vi "uServices Status Check.vi"(8 "error in (no error)":errorcluster, 11 "Guardian in":refnum<class "Guardian.lvclass">) -> (0 "error out":errorcluster, 3 "Guardian out":refnum<class "Guardian.lvclass">)   [LabVIEW 2026, in "TALOS.lvlib" / "Guardian.lvlib" / "Guardian.lvclass"]
uses:
  Guardian.lvclass
  C:/LabVIEW Code/TALOS/builds/Actor Framework PPL/Actor Framework.lvlibp/1abvi3w/vi.lib/ActorFramework/Actor/Actor.lvclass
  Ancestor/Ancestor/Ancestor.lvclass/Ancestor.ctl
  Classes/Speedometer/Speedometer.lvclass/Speedometer.ctl
  Classes/uService List/uService List.lvclass/uService List.ctl
  Guardian Messages/uService not responding Msg/uService not responding Msg.lvclass/uService not responding Msg.ctl
  Classes/uService List/Get all IDs.vi
  Classes/uService List/Get Last Pat.vi
  Support VIs/Generate Error.vi
  <vilib>/Utility/High Resolution Relative Seconds.vi
  FGV/Error Memory/Get Error Description.vi
  Support VIs/Get PC name.vi
  Ancestor/Ancestor/Read ID.vi
  Support VIs/Get Class Name.vi
  FGV/Error Memory/Error Memory Core.vi
  <vilib>/AdvancedString/Delimited String to 1D String Array.vi
  <vilib>/AdvancedString/Delimited String to 1D String Array (string).vi
  Support VIs/Circus Root Path.vi
  FGV/Error Memory/Error Crt Lvl checker.vi
  FGV/Error Memory/Error Memory Core.vi/40c8088d-b597-4017-91af-faa98e00292e.vi
  FGV/Error Memory/Error Memory Core.vi/d4a3ab98-063c-4e44-b43d-fbdcfe6c2be2.vi
  Support VIs/Global Memory.vi
  <vilib>/Utility/LVClass/Get LV Class Name.vi
  Support VIs/Is in Packed Library.vi
  Support VIs/TALOS Root path.vi
  Support VIs/Read CSV worksheet.vi
  Support VIs/Global Constants.vi
  <vilib>/Utility/error.llb/General Error Handler.vi
  <vilib>/Utility/config.llb/Open Config Data.vi
  <vilib>/Utility/config.llb/Get Section Names.vi
  <vilib>/Utility/config.llb/Get Key Names.vi
  <vilib>/Utility/config.llb/Read Key.vi
  <vilib>/Utility/config.llb/Read Key (String).vi
  <vilib>/Utility/config.llb/Close Config Data.vi
  builds/Actor Framework PPL/Actor Framework.lvlibp/1abvi3w/vi.lib/ActorFramework/Message Enqueuer/Enqueue.vi
  Support VIs/Error Log.vi
  Support VIs/System Log.vi
  Ancestor/Ancestor/Ancestor.lvclass
  <vilib>/Comparison/Equal/Equal Functor/Equal Functor.lvclass
  Classes/Speedometer/Speedometer.lvclass
  Guardian Messages/uService not responding Msg/uService not responding Msg.lvclass
  TALOS.lvlib
  Classes/uService List/uService List.lvclass
  builds/Actor Framework PPL/Actor Framework.lvlibp/1abvi3w/vi.lib/ActorFramework/Actor/Actor.lvclass
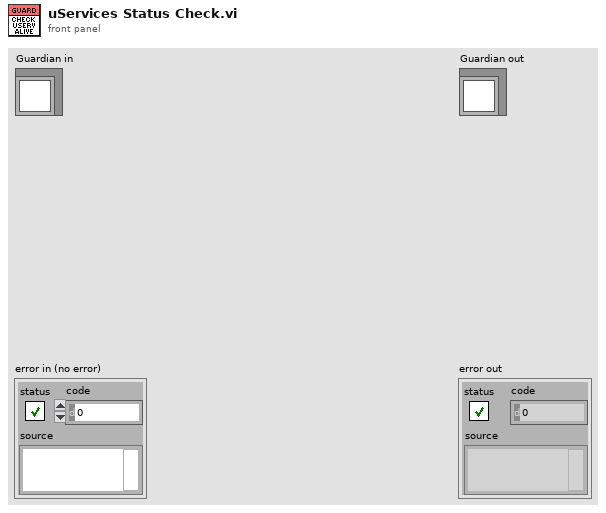
[diagram p1: front panel]
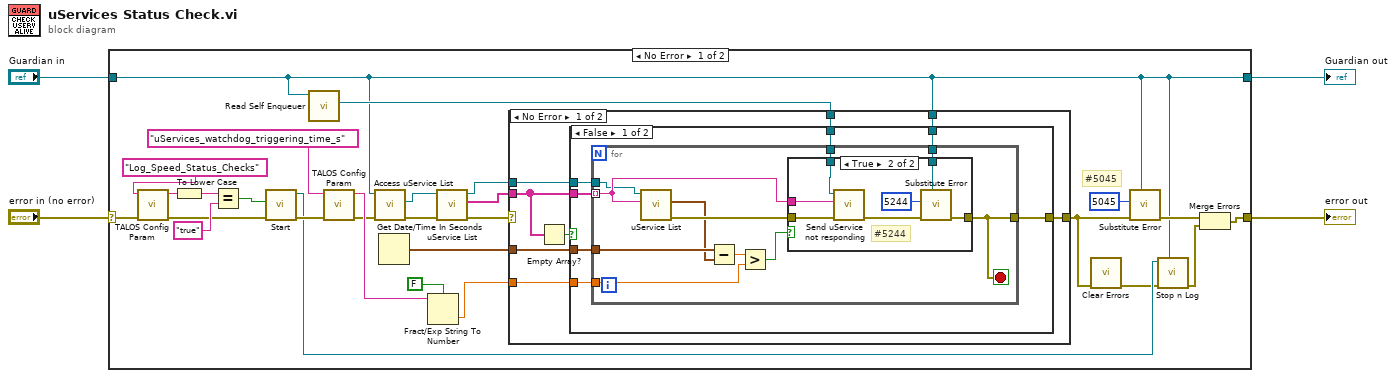
[diagram p0: block diagram]
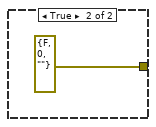
[diagram p3: hidden frame]
diagram:
  n1 = case shown="No Error" "error in (no error)" {
    selector: "error in (no error)" -> [w16 w70]
    tunnel: [w9 w70] -> w2
    tunnel: [w5 w69] -> w1
    tunnel: "Guardian in" -> [w5 w69]
    frame No Error {
      # "#5045"
      n2 = call "TALOS Config Param.vi"("error in (no error)"=w16, "Parameter Name"="Log_Speed_Status_Checks") -> ("error out"=w15:errorcluster, "Output"=w20:string)  [unwired: 8 in]
      n3 = To Lower Case(string=w20) -> (all lower case string=w19:string)
      n4 = Equal?(x=w19, y="true") -> (x = y?=w14:bool)
      n5 = call "Start.vi"("error in (no error)"=w15, "Active?"=w14) -> ("error out"=w13:errorcluster, "Speedometer out"=w12:refnum<class "Speedometer.lvclass">)  [unwired: 8 in]
      n6 = call "Read Self Enqueuer.vi"("Actor"=w5) -> ("Self Enqueuer"=w31:refnum<class "Message Enqueuer.lvclass">)  [unwired: 10 in]
      n7 = call "TALOS Config Param.vi"("error in (no error)"=w13, "Parameter Name"="uServices_watchdog_triggering_time_s") -> ("error out"=w23:errorcluster, "Output"=w28:string)  [unwired: 8 in]
      n8 = call-dynamic "Access uService List.vi"("error in (no error)"=w23, "Ancestor in"=w5) -> ("error out"=w25:errorcluster, "uService List out"=w24:refnum<class "uService List.lvclass">)  [unwired: 7 in, 1 out]
      n9 = Get Date/Time In Seconds() -> (seconds since 1Jan1904=w32:timestamp)
      n10 = Fract/Exp String To Number(use system decimal point (T)=FALSE, string=w28) -> (number=w27:dbl)  [unwired: 2 in, 1 out]
      n11 = call-poly "uService List.vi"("error in (no error)"=w25, "uService List"=w24) -> ("error out"=w29:errorcluster, "All IDs"=w22:string[], "uService List out"=w21:refnum<class "uService List.lvclass">)  [unwired: 7 in]
      n12 = case shown="No Error" w29 {
        selector: w29 -> [_ w68]
        tunnel: w32 -> [w40 _]
        tunnel: w31 -> [w39 _]
        tunnel: w27 -> [w38 _]
        tunnel: [w37 w68] -> w7
        tunnel: w22 -> [w35 _]
        tunnel: w21 -> [w34 _]
        tunnel: w5 -> [w33 _]
        frame No Error {
          n13 = Empty Array?(array=w35) -> (empty?=w36:bool)
          n14 = case shown="False" w36 {
            tunnel: w40 -> [w47 _]
            tunnel: w39 -> [w46 _]
            tunnel: w35 -> [w45 _]
            tunnel: w38 -> [w44 _]
            tunnel: [w42 errorcluster {"status"=FALSE, "code"=0, "source"=""} ("error out")] -> w37
            tunnel: w34 -> [w43 _]
            tunnel: w33 -> [w41 _]
            frame False {
              n15 = for {
                tunnel: w45 -> [w52] mode=indexing
                tunnel: w47 -> [w58]
                tunnel: w46 -> [w56]
                tunnel: w44 -> [w54]
                tunnel: w43 -> [w51]
                tunnel: [w49] -> w42
                tunnel: w41 -> [w48]
                stop <- w49 stop-if-true
                n16 = call-poly "uService List.vi"("ID"=w52, "uService List in"=w51) -> ("error out"=w53:errorcluster, "Last Pat"=w50:timestamp)  [unwired: 7 in, 1 out]
                n17 = Subtract(x=w58, y=w50) -> (x-y=w57:dbl)
                n18 = Greater?(x=w57, y=w54) -> (0:w55:bool)
                n19 = case shown="True" w55 {
                  tunnel: w56 -> [_ w64]
                  tunnel: w52 -> [_ w65]
                  tunnel: w53 -> [w59 w66]
                  tunnel: [w59 w61] -> w49
                  tunnel: w48 -> [_ w60]
                  frame False {
                  }
                  frame True {
                    # "#5244"
                    n20 = call "Send uService not responding.vi"("error in (no error)"=w66, "uService"=w65, "Message Enqueuer"=w64) -> ("error out"=w62:errorcluster)  [unwired: 7 in, 1 out]
                    n21 = call "Substitute Error.vi"("LabVIEW Object"=w60, "error in (no error)"=w62, "Error Code"=5244) -> ("error out"=w61:errorcluster)  [unwired: 8 in]
                  }
                }
              }
            }
            frame True {
            }
          }
        }
        frame Error {
        }
      }
      n22 = call <vilib>:"Clear Errors.vi"("error in (no error)"=w7) -> ("error out"=w10:errorcluster)  [unwired: 5 in, 1 out]
      n23 = call "Substitute Error.vi"("LabVIEW Object"=w5, "error in (no error)"=w7, "Error Code"=5045) -> ("error out"=w6:errorcluster)  [unwired: 8 in]
      n24 = call "Stop n Log.vi"("Object in"=w5, "error in (no error)"=w10, "Speedometer in"=w12) -> ("error out"=w11:errorcluster)  [unwired: 8 in]
      n25 = Merge Errors(w6, w11) -> (w9:errorcluster)
    }
    frame Error {
    }
  }
  "error out" <- w2
  "Guardian out" <- w1
